vi "Receive DBL.vi"(8 "error in (no error)":errorcluster, 10 "Broadcast DBL Msg":refnum<class "Broadcast DBL Msg.lvclass">, 11 "IViewable In":refnum<class "IViewable.lvclass">) -> (0 "error out":errorcluster, 3 "IViewable Out":refnum<class "IViewable.lvclass">)   [LabVIEW 2015, in "IViewable.lvlib" / "IViewable.lvclass"]
uses:
  IViewable.lvclass
  IViewable Messages/Broadcast DBL Msg/Broadcast DBL Msg.lvclass
  <vilib>/ActorFramework/Actor/Actor.lvclass/Actor.ctl
  <vilib>/ActorFramework/Actor/Actor.lvclass
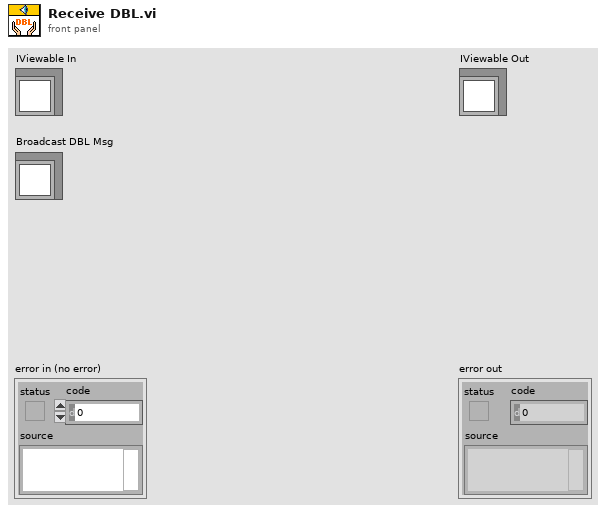
[diagram p1: front panel]
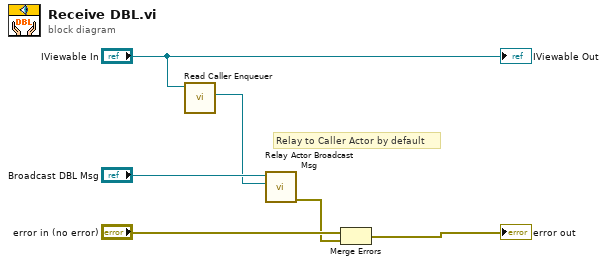
[diagram p0: block diagram]
diagram:
  # "Relay to Caller Actor by default"
  n1 = call <vilib>:"Read Caller Enqueuer.vi"("Actor"="IViewable In") -> ("Caller Enqueuer"=w3:refnum<class "Message Enqueuer.lvclass">)  [unwired: 10 in]
  n2 = call-dynamic "Relay Actor Broadcast Msg.vi"("Caller Enqueuer"=w3, "ActorEventMessage In"="Broadcast DBL Msg") -> ("error out"=w1:errorcluster)  [unwired: 9 in]
  n3 = Merge Errors("error in (no error)", w1) -> (→"error out":errorcluster)
  "IViewable Out" <- "IViewable In"
